vi "Parse.vi"(8 "error in":errorcluster, 11 "reference in":refnum<class "Electronic Datasheet.lvclass">) -> (0 "error out":errorcluster, 3 "reference out":refnum<class "Electronic Datasheet.lvclass">)   [LabVIEW 2024, in "Electronic Datasheet.lvlib" / "Electronic Datasheet.lvclass"]
uses:
  Electronic Datasheet/Electronic Datasheet.lvclass
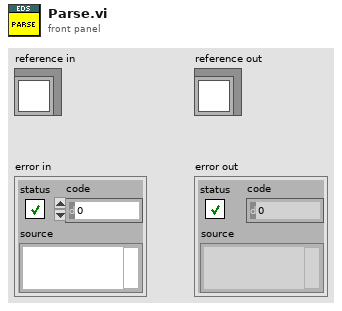
[diagram p1: front panel]
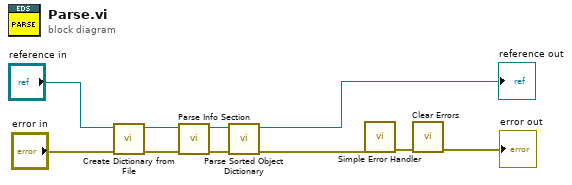
[diagram p0: block diagram]
diagram:
  n1 = call "Create Dictionary from File.vi"("error in"="error in", "reference in"="reference in") -> ("error out"=w6:errorcluster, "reference out"=w5:refnum<class "Electronic Datasheet.lvclass">)  [unwired: 8 in]
  n2 = call "Parse Info Section.vi"("error in"=w6, "reference in"=w5) -> ("error out"=w3:errorcluster, "reference out"=w4:refnum<class "Electronic Datasheet.lvclass">)  [unwired: 8 in]
  n3 = call "Parse Sorted Object Dictionary.vi"("error in"=w3, "reference in"=w4) -> ("error out"=w2:errorcluster, "reference out"=→"reference out":refnum<class "Electronic Datasheet.lvclass">)  [unwired: 8 in]
  n4 = call <vilib>:"Simple Error Handler.vi"("error in (no error)"=w2) -> ("error out"=w9:errorcluster)  [unwired: 4 in, 4 out]
  n5 = call <vilib>:"Clear Errors.vi"("error in (no error)"=w9) -> ("error out"=→"error out":errorcluster)  [unwired: 5 in, 1 out]
